vi "AutonomousMain.vi"() -> (0 "Terminate":bool)   [LabVIEW 2015]
uses:
  <vilib>/Rock Robotics/WPI/DriverStation/WPI_DriverStationRobotMode2.ctl
  <vilib>/Rock Robotics/WPI/CAN/TalonSRX/WPI_CANTalonSRX_APIControlMode.ctl
  <vilib>/Rock Robotics/WPI/Solenoid/WPI_SolenoidValue.ctl
  Utilities/AutoVars.vi
  Utilities/MotorPositionGlobals.vi
  Utilities/GlobalVisionVars.vi
  Utilities/VisionGlobals.vi
  <vilib>/Rock Robotics/WPI/Solenoid/WPI_SolenoidSetEnum.vi
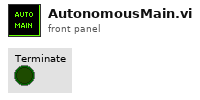
[diagram p1: front panel]
types:
  T1 = enum16{"WaitingForInput", "Driving", "TurnToTarget", "DriveMore", "Shoot", "End"}
  T2 = typedef "WPI_DriverStationRobotMode2.ctl" = enum16{"Autonomous Disabled", "Autonomous Enabled", "Teleop Disabled", "Teleop Enabled", "Disconnected", "Finish", "Test Disabled", "Test Enabled", "Emergency Stopped"}
  T3 = enum16{"Far Left", "Pos 2", "Pos 3", "Pos 4", "Far Right"}
  T4 = typedef "WPI_SolenoidValue.ctl" = enum16{"Off", "On", "Forward", "Reverse"}
  T5 = typedef "WPI_MotorControlDeviceRef.ctl" = cluster{"DeviceStatus":errorcluster, "Type":T6, "PWM":cluster{"PWM Channel":T7, "DeadBand":T8}, "CAN":cluster{"Device Number":u8, "Control Mode":T9, "Semaphore":T10, "Max Vout":dbl, "TalonSRX Control Mode":T11}, "Invert":bool}
  T6 = typedef "WPI_MotorControlType.ctl" = enum16{"PWM", "CAN", "CANTalonSRX"}
  T7 = typedef "FPGA_DIOPWMChannel.ctl" = enum8{"PWM 0", "PWM 1", "PWM 2", "PWM 3", "PWM 4", "PWM 5", "PWM 6", "PWM 7", "PWM 8", "PWM 9", "PWM MXP 0", "PWM MXP 1", "PWM MXP 2", "PWM MXP 3", "PWM MXP 4", "PWM MXP 5", "PWM MXP 6", "PWM MXP 7", "PWM MXP 8", "PWM MXP 9", "Invalid"}
  T8 = typedef "WPI_PWMDeadband.ctl" = cluster{"Name":string, "maxPositivePwm":i32, "minPositivePwm":i32, "centerPwm":i32, "maxNegativePwm":i32, "minNegativePwm":i32, "angularRange":u16}
  T9 = typedef "WPI_CANJaguar_ControlMode.ctl" = enum8{"Percent VBus", "Current", "Speed", "Position", "Voltage"}
  T10 = typedef "Semaphore RefNum" = refnum<k1>
  T11 = typedef "WPI_CANTalonSRX_APIControlMode.ctl" = enum8{"Percent VBus", "Speed", "Position", "Slave", "Unchanged / Invalid", "Voltage Compensation", "Current", "Motion Profile"}
  T12 = typedef "WPI_DigitalOutputDevRef.ctl" = cluster{"DIO Channel":T13, "DevStatus":errorcluster}
  T13 = typedef "FPGA_DIOChannel.ctl" = enum8{"DIO 0", "DIO 1", "DIO 2", "DIO 3", "DIO 4", "DIO 5", "DIO 6", "DIO 7", "DIO 8", "DIO 9", "DIO MXP 0", "DIO MXP 1", "DIO MXP 2", "DIO MXP 3", "DIO MXP 4", "DIO MXP 5", "DIO MXP 6", "DIO MXP 7", "DIO MXP 8", "DIO MXP 9", "DIO MXP 10", "DIO MXP 11", "DIO MXP 12", "DIO MXP 13", "DIO MXP 14", "DIO MXP 15", "Invalid"}
  T14 = typedef "WPI_GyroDevRef.ctl" = cluster{"DevStatus":errorcluster, "Analog Channel":T15, "Offset":dbl, "Gain (VoltsPerDegree/Second)":dbl, "Gyro Type":enum16{"Analog", "XRS450"}, "Handle":i32, "SPI Bus":T16, "Device Found":bool, "Sample Rate":dbl, "Calibrate On Open":bool}
  T15 = typedef "FPGA_AIChannel.ctl" = enum8{"AI 0", "AI 1", "AI 2", "AI 3", "AI MXP 0", "AI MXP 1", "AI MXP 2", "AI MXP 3", "Invalid"}
  T16 = typedef "spi_bus.ctl" = enum16{"SPI On-Board, CS0", "SPI On-Board, CS1", "SPI On-Board, CS2", "SPI On-Board, CS3", "SPI MXP", "Invalid"}
  T17 = typedef "WPI_SolenoidDevRef.ctl" = cluster{"DevStatus":errorcluster, "Pneumatics Control Module":u8, "Forward Solenoid Channel":T18, "Reverse Solenoid Channel":T18}
  T18 = typedef "WPI_SolenoidChannel.ctl" = enum8{"Solenoid 0", "Solenoid 1", "Solenoid 2", "Solenoid 3", "Solenoid 4", "Solenoid 5", "Solenoid 6", "Solenoid 7", "Invalid"}
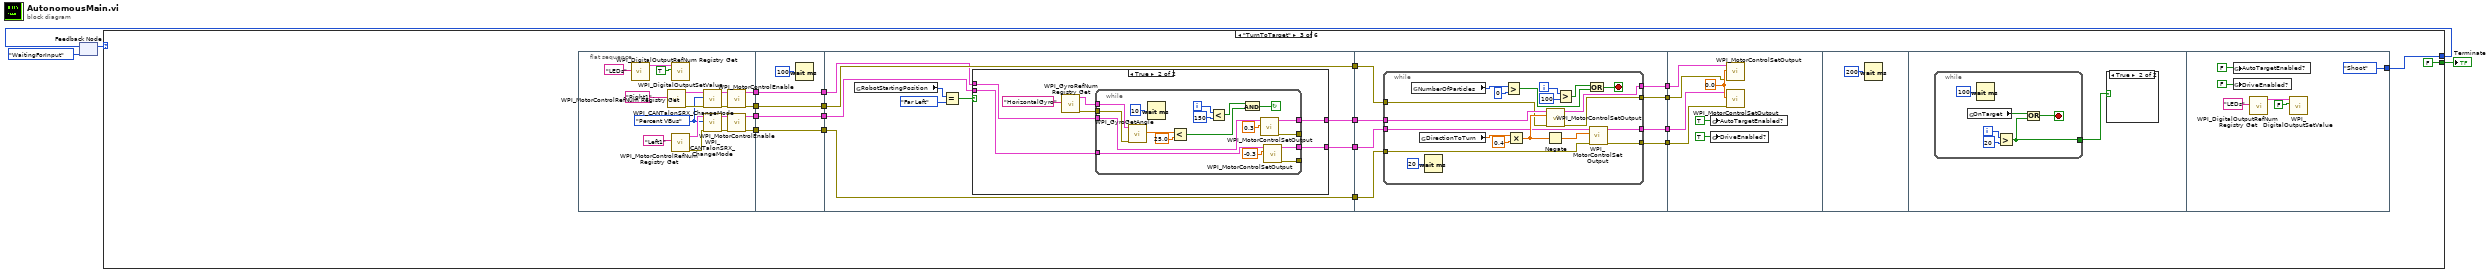
[diagram p0: block diagram]
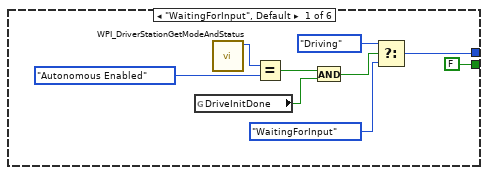
[diagram p2: hidden frame]
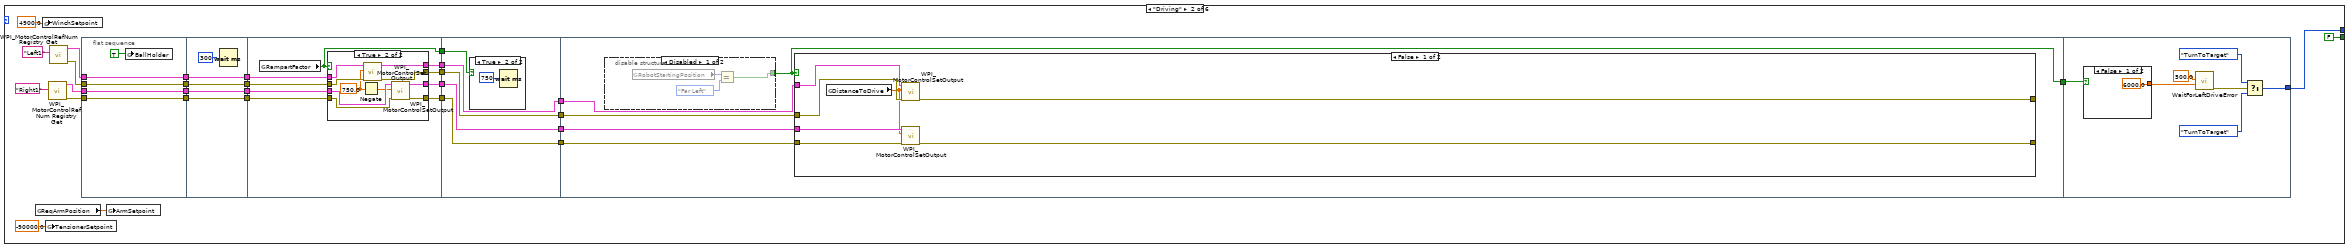
[diagram p3: hidden frame]
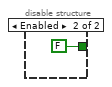
[diagram p6: hidden frame]
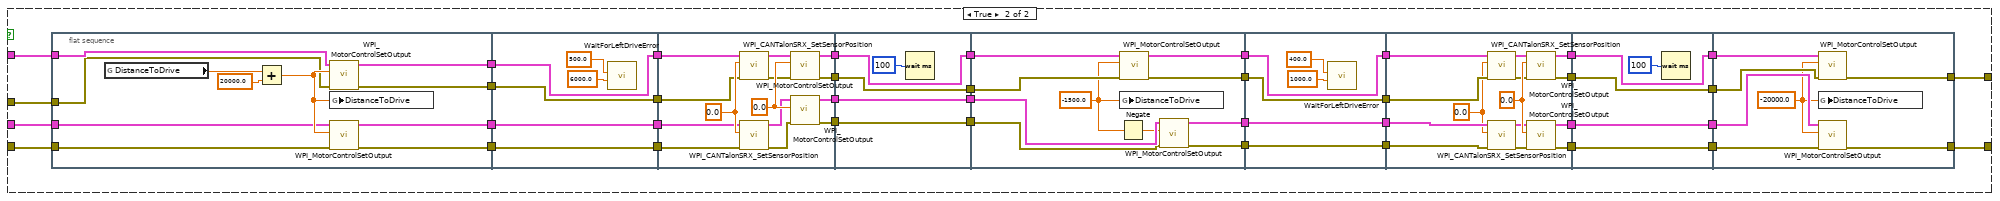
[diagram p7: hidden frame]
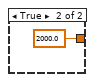
[diagram p8: hidden frame]
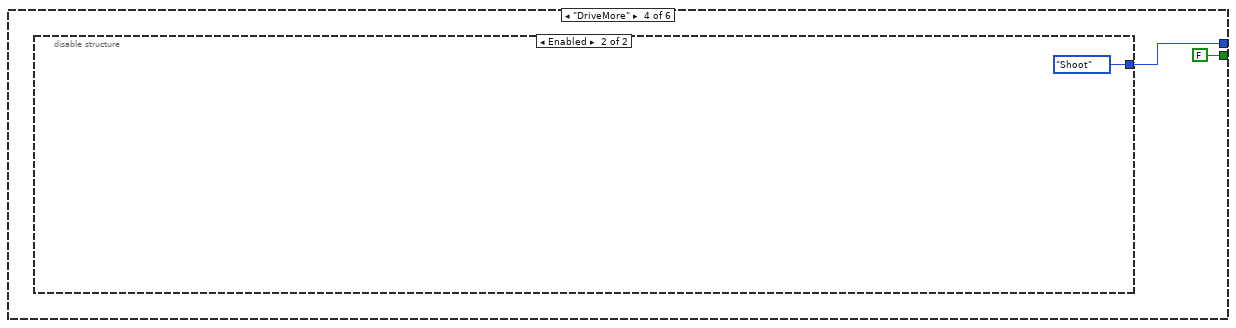
[diagram p11: hidden frame]
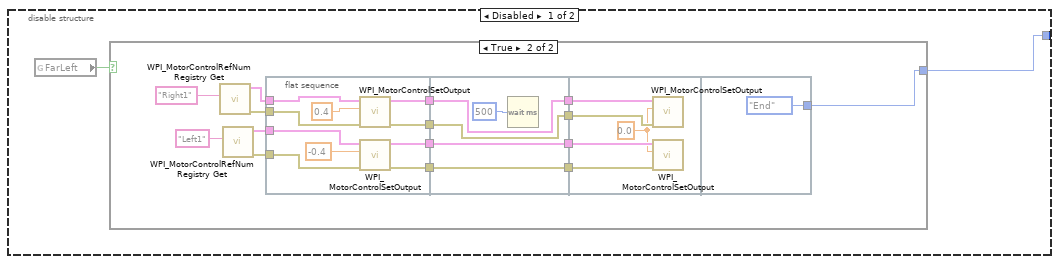
[diagram p12: hidden frame]
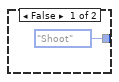
[diagram p13: hidden frame]
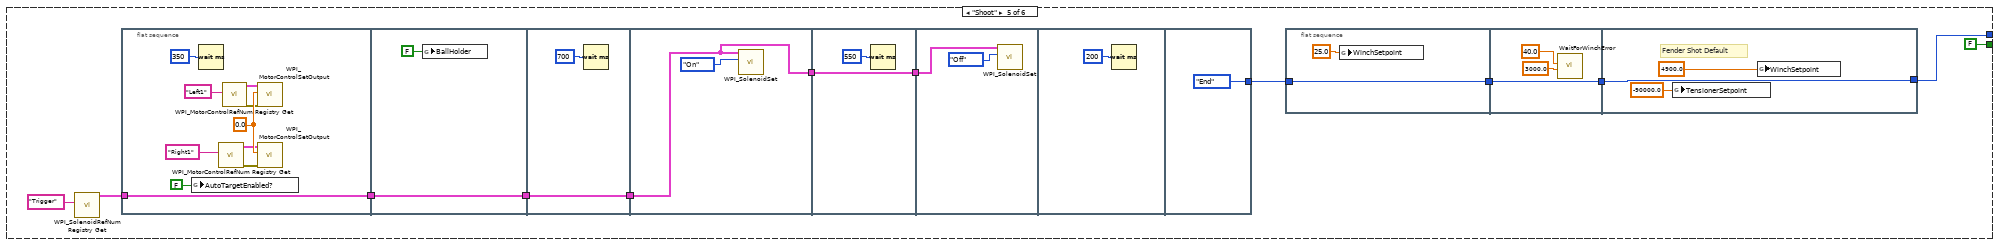
[diagram p14: hidden frame]
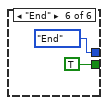
[diagram p15: hidden frame]
diagram:
  n1 = feedback #1(T1."WaitingForInput" ("AutoStateMachine")) -> (w1:T1)
  n2 = case shown="\"TurnToTarget\"" w1 {
    tunnel: [w13 w25 w240 w350 w393 T1."End" ("AutoStateMachine")] -> w4
    tunnel: [FALSE FALSE FALSE FALSE FALSE TRUE] -> w3
    frame "WaitingForInput", Default {
      n3 = global read "AutoVars.vi" "DriveInitDone"() -> (w8:bool)
      n4 = call <vilib>:"WPI_DriverStationGetModeAndStatus.vi"() -> ("Robot Mode"=w11:T2)  [unwired: 10 in, 1 out]
      n5 = Equal?(x=w11, y=WPI_DriverStationRobotMode2."Autonomous Enabled" ("Robot Mode")) -> (x = y?=w9:bool)
      n6 = And(x=w9, y=w8) -> (x .and. y?=w7:bool)
      n7 = Select(t=T1."Driving" ("AutoStateMachine"), s=w7, f=T1."WaitingForInput" ("AutoStateMachine")) -> (s? t:f=w13:T1)
    }
    frame "Driving" {
      n8 = global read "AutoVars.vi" "ReqArmPosition"() -> (w24:dbl)
      n9 = global write "MotorPositionGlobals.vi" "WinchSetpoint"(4900.0 ("WinchSetpoint")) -> ()
      n10 = global write "MotorPositionGlobals.vi" "TensionerSetpoint"(-90000.0 ("TensionerSetpoint")) -> ()
      n11 = call <vilib>:"WPI_MotorControlRefNum Registry Get.vi"("refnum name"="Right1") -> ("error out"=w36:errorcluster, "MotorControlDevRef"=w37:T5)  [unwired: 9 in]
      n12 = call <vilib>:"WPI_MotorControlRefNum Registry Get.vi"("refnum name"="Left1") -> ("error out"=w34:errorcluster, "MotorControlDevRef"=w35:T5)  [unwired: 9 in]
      n13 = flat-sequence {
        tunnel: w34 -> [w44]
        tunnel: w35 -> [w45]
        tunnel: w36 -> [w46]
        tunnel: w37 -> [w47]
        tunnel: [w47] -> w23
        tunnel: [w46] -> w21
        tunnel: [w45] -> w19
        tunnel: [w44] -> w17
        tunnel: w23 -> [w52]
        tunnel: [w52] -> w22
        tunnel: w21 -> [w51]
        tunnel: [w51] -> w20
        tunnel: w19 -> [w50]
        tunnel: [w50] -> w18
        tunnel: w17 -> [w49]
        tunnel: [w49] -> w16
        tunnel: [w57] -> w33
        tunnel: [w56] -> w31
        tunnel: [w55] -> w29
        tunnel: [w54] -> w27
        tunnel: w22 -> [w61]
        tunnel: w20 -> [w60]
        tunnel: w18 -> [w59]
        tunnel: w16 -> [w58]
        tunnel: [w53] -> w15
        tunnel: w33 -> [w80]
        tunnel: [w80] -> w32
        tunnel: w31 -> [w79]
        tunnel: [w79] -> w30
        tunnel: w29 -> [w78]
        tunnel: [w78] -> w28
        tunnel: w27 -> [w77]
        tunnel: [w77] -> w26
        tunnel: w15 -> [w76]
        tunnel: w32 -> [w86]
        tunnel: w30 -> [w85]
        tunnel: w28 -> [w83]
        tunnel: w26 -> [w84]
        tunnel: [w82] -> w14
        tunnel: [w215] -> w25
        tunnel: w14 -> [w214]
        frame #0 {
          n14 = global write "MotorPositionGlobals.vi" "BallHolder"(TRUE ("BallHolder")) -> ()
        }
        frame #1 {
          n15 = Wait (ms)(milliseconds to wait=u32 300) -> ()  [unwired: 1 out]
        }
        frame #2 {
          n16 = global read "AutoVars.vi" "RampartFactor"() -> (w53:bool)
          n17 = case shown="True" w53 {
            tunnel: w61 -> [w63 w75]
            tunnel: w60 -> [w62 w74]
            tunnel: w59 -> [w65 w73]
            tunnel: w58 -> [w64 w72]
            tunnel: [w63 w71] -> w57
            tunnel: [w62 w70] -> w56
            tunnel: [w65 w69] -> w55
            tunnel: [w64 w68] -> w54
            frame False {
            }
            frame True {
              w67 = 750.0
              n18 = Negate(x=w67) -> (-x=w66:dbl)
              n19 = call <vilib>:"WPI_MotorControlSetOutput.vi"("error in (no error)"=w72, "Output"=w67, "MotorControlDevRef"=w73) -> ("error out"=w68:errorcluster, "MotorControlDevRef"=w69:T5)  [unwired: 6 in, 1 out]
              n20 = call <vilib>:"WPI_MotorControlSetOutput.vi"("error in (no error)"=w74, "Output"=w66, "MotorControlDevRef"=w75) -> ("error out"=w70:errorcluster, "MotorControlDevRef"=w71:T5)  [unwired: 6 in, 1 out]
            }
          }
        }
        frame #3 {
          n21 = case shown="True" w76 {
            frame False {
            }
            frame True {
              n22 = Wait (ms)(milliseconds to wait=u32 750) -> ()  [unwired: 1 out]
            }
          }
        }
        frame #4 {
          n23 = disable-structure shown="Disabled" {
            disable-tunnel: [w87 FALSE] -> w82
            frame Disabled {
              n24 = global read "AutoVars.vi" "RobotStartingPosition"() -> (w89:T3)
              n25 = Equal?(x=w89, y=T3."Far Left") -> (x = y?=w87:bool)
            }
            frame Enabled {
            }
          }
          n26 = case shown="False" w82 {
            tunnel: w86 -> [w97 w134]
            tunnel: w85 -> [w96 w132]
            tunnel: w84 -> [w95 w133]
            tunnel: w83 -> [w93 w135]
            tunnel: [w92 w115] -> _
            tunnel: [w91 w114] -> _
            frame False {
              n27 = global read "AutoVars.vi" "DistanceToDrive"() -> (w94:dbl)
              n28 = call <vilib>:"WPI_MotorControlSetOutput.vi"("error in (no error)"=w95, "Output"=w94, "MotorControlDevRef"=w93) -> ("error out"=w92:errorcluster)  [unwired: 6 in, 2 out]
              n29 = call <vilib>:"WPI_MotorControlSetOutput.vi"("error in (no error)"=w96, "Output"=w94, "MotorControlDevRef"=w97) -> ("error out"=w91:errorcluster)  [unwired: 6 in, 2 out]
            }
            frame True {
              n30 = flat-sequence {
                tunnel: w135 -> [w143]
                tunnel: w134 -> [w142]
                tunnel: w133 -> [w141]
                tunnel: w132 -> [w140]
                tunnel: [w139] -> w130
                tunnel: [w138] -> w128
                tunnel: [w137] -> w126
                tunnel: [w136] -> w125
                tunnel: [w150] -> w131
                tunnel: w130 -> [w150]
                tunnel: [w149] -> w129
                tunnel: w128 -> [w149]
                tunnel: [w148] -> w127
                tunnel: w126 -> [w148]
                tunnel: w125 -> [w147]
                tunnel: [w147] -> w124
                tunnel: w131 -> [w160]
                tunnel: w129 -> [w159]
                tunnel: w127 -> [w158]
                tunnel: w124 -> [w157]
                tunnel: [w156] -> w113
                tunnel: [w155] -> w111
                tunnel: [w154] -> w109
                tunnel: [w153] -> w107
                tunnel: w113 -> [w171]
                tunnel: [w171] -> w112
                tunnel: w111 -> [w170]
                tunnel: [w170] -> w110
                tunnel: w109 -> [w169]
                tunnel: [w169] -> w108
                tunnel: w107 -> [w168]
                tunnel: [w168] -> w106
                tunnel: w112 -> [w181]
                tunnel: w110 -> [w180]
                tunnel: w108 -> [w179]
                tunnel: w106 -> [w178]
                tunnel: [w177] -> w123
                tunnel: [w176] -> w121
                tunnel: [w175] -> w119
                tunnel: [w174] -> w117
                tunnel: w123 -> [w187]
                tunnel: [w187] -> w122
                tunnel: w121 -> [w186]
                tunnel: [w186] -> w120
                tunnel: w119 -> [w185]
                tunnel: [w185] -> w118
                tunnel: w117 -> [w184]
                tunnel: [w184] -> w116
                tunnel: w122 -> [w200]
                tunnel: w120 -> [w199]
                tunnel: w118 -> [w198]
                tunnel: w116 -> [w197]
                tunnel: [w195] -> w99
                tunnel: [w194] -> w101
                tunnel: [w193] -> w103
                tunnel: [w192] -> w105
                tunnel: w105 -> [w206]
                tunnel: [w206] -> w104
                tunnel: w103 -> [w205]
                tunnel: [w205] -> w102
                tunnel: w101 -> [w204]
                tunnel: [w204] -> w100
                tunnel: w99 -> [w203]
                tunnel: [w203] -> w98
                tunnel: w104 -> [w210]
                tunnel: w102 -> [w211]
                tunnel: w100 -> [w212]
                tunnel: w98 -> [w213]
                tunnel: [w209] -> w115
                tunnel: [w208] -> w114
                frame #0 {
                  n31 = global read "AutoVars.vi" "DistanceToDrive"() -> (w145:dbl)
                  n32 = Add(x=w145, y=20000.0) -> (x+y=w144:dbl)
                  n33 = call <vilib>:"WPI_MotorControlSetOutput.vi"("error in (no error)"=w141, "Output"=w144, "MotorControlDevRef"=w143) -> ("error out"=w138:errorcluster, "MotorControlDevRef"=w139:T5)  [unwired: 6 in, 1 out]
                  n34 = global write "AutoVars.vi" "DistanceToDrive"(w144) -> ()
                  n35 = call <vilib>:"WPI_MotorControlSetOutput.vi"("error in (no error)"=w140, "Output"=w144, "MotorControlDevRef"=w142) -> ("error out"=w136:errorcluster, "MotorControlDevRef"=w137:T5)  [unwired: 6 in, 1 out]
                }
                frame #1 {
                  n36 = call "WaitForLeftDriveError.vi"("Timeout (ms)"=6000.0, "AllowedError"=500.0) -> ()  [unwired: 9 in, 1 out]
                }
                frame #2 {
                  w165 = 0.0 ("New Sensor Position")
                  w166 = 0.0 ("Output")
                  n37 = call <vilib>:"WPI_CANTalonSRX_SetSensorPosition.vi"("error in (no error)"=w159, "New Sensor Position"=w165, "CAN Talon SRX Ref"=w160) -> ("error out"=w163:errorcluster, "CAN Talon SRX Ref"=w164:T5)  [unwired: 7 in]
                  n38 = call <vilib>:"WPI_CANTalonSRX_SetSensorPosition.vi"("error in (no error)"=w157, "New Sensor Position"=w165, "CAN Talon SRX Ref"=w158) -> ("error out"=w161:errorcluster, "CAN Talon SRX Ref"=w162:T5)  [unwired: 7 in]
                  n39 = call <vilib>:"WPI_MotorControlSetOutput.vi"("error in (no error)"=w163, "Output"=w166, "MotorControlDevRef"=w164) -> ("error out"=w155:errorcluster, "MotorControlDevRef"=w156:T5)  [unwired: 6 in, 1 out]
                  n40 = call <vilib>:"WPI_MotorControlSetOutput.vi"("error in (no error)"=w161, "Output"=w166, "MotorControlDevRef"=w162) -> ("error out"=w153:errorcluster, "MotorControlDevRef"=w154:T5)  [unwired: 6 in, 1 out]
                }
                frame #3 {
                  n41 = Wait (ms)(milliseconds to wait=u32 100) -> ()  [unwired: 1 out]
                }
                frame #4 {
                  w172 = -1500.0
                  n42 = Negate(x=w172) -> (-x=w173:dbl)
                  n43 = call <vilib>:"WPI_MotorControlSetOutput.vi"("error in (no error)"=w180, "Output"=w172, "MotorControlDevRef"=w181) -> ("error out"=w176:errorcluster, "MotorControlDevRef"=w177:T5)  [unwired: 6 in, 1 out]
                  n44 = global write "AutoVars.vi" "DistanceToDrive"(w172) -> ()
                  n45 = call <vilib>:"WPI_MotorControlSetOutput.vi"("error in (no error)"=w178, "Output"=w173, "MotorControlDevRef"=w179) -> ("error out"=w174:errorcluster, "MotorControlDevRef"=w175:T5)  [unwired: 6 in, 1 out]
                }
                frame #5 {
                  n46 = call "WaitForLeftDriveError.vi"("Timeout (ms)"=1000.0, "AllowedError"=400.0) -> ()  [unwired: 9 in, 1 out]
                }
                frame #6 {
                  w196 = 0.0 ("New Sensor Position")
                  w201 = 0.0 ("Output")
                  n47 = call <vilib>:"WPI_CANTalonSRX_SetSensorPosition.vi"("error in (no error)"=w199, "New Sensor Position"=w196, "CAN Talon SRX Ref"=w200) -> ("error out"=w190:errorcluster, "CAN Talon SRX Ref"=w191:T5)  [unwired: 7 in]
                  n48 = call <vilib>:"WPI_CANTalonSRX_SetSensorPosition.vi"("error in (no error)"=w197, "New Sensor Position"=w196, "CAN Talon SRX Ref"=w198) -> ("error out"=w188:errorcluster, "CAN Talon SRX Ref"=w189:T5)  [unwired: 7 in]
                  n49 = call <vilib>:"WPI_MotorControlSetOutput.vi"("error in (no error)"=w190, "Output"=w201, "MotorControlDevRef"=w191) -> ("error out"=w194:errorcluster, "MotorControlDevRef"=w195:T5)  [unwired: 6 in, 1 out]
                  n50 = call <vilib>:"WPI_MotorControlSetOutput.vi"("error in (no error)"=w188, "Output"=w201, "MotorControlDevRef"=w189) -> ("error out"=w192:errorcluster, "MotorControlDevRef"=w193:T5)  [unwired: 6 in, 1 out]
                }
                frame #7 {
                  n51 = Wait (ms)(milliseconds to wait=u32 100) -> ()  [unwired: 1 out]
                }
                frame #8 {
                  w207 = -20000.0 ("Output")
                  n52 = call <vilib>:"WPI_MotorControlSetOutput.vi"("error in (no error)"=w212, "Output"=w207, "MotorControlDevRef"=w213) -> ("error out"=w209:errorcluster)  [unwired: 6 in, 2 out]
                  n53 = global write "AutoVars.vi" "DistanceToDrive"(w207) -> ()
                  n54 = call <vilib>:"WPI_MotorControlSetOutput.vi"("error in (no error)"=w210, "Output"=w207, "MotorControlDevRef"=w211) -> ("error out"=w208:errorcluster)  [unwired: 6 in, 2 out]
                }
              }
            }
          }
        }
        frame #5 {
          n55 = case shown="False" w214 {
            tunnel: [6000.0 ("Timeout (ms)") 2000.0 ("Timeout (ms)")] -> w220
            frame False {
            }
            frame True {
            }
          }
          n56 = call "WaitForLeftDriveError.vi"("Timeout (ms)"=w220, "AllowedError"=500.0) -> ("error out"=w218:errorcluster)  [unwired: 9 in]
          n57 = Select(t=T1."TurnToTarget", s=w218, f=T1."TurnToTarget" ("AutoStateMachine")) -> (s? t:f=w215:T1)
        }
      }
      n58 = global write "MotorPositionGlobals.vi" "ArmSetpoint"(w24) -> ()
    }
    frame "TurnToTarget" {
      n59 = flat-sequence {
        tunnel: [w247] -> w238
        tunnel: [w246] -> w237
        tunnel: [w245] -> w236
        tunnel: [w244] -> w235
        tunnel: w238 -> [w260]
        tunnel: w237 -> [w259]
        tunnel: w236 -> [w262]
        tunnel: w235 -> [w261]
        tunnel: [w262] -> w230
        tunnel: [w261] -> w228
        tunnel: [w260] -> w226
        tunnel: [w259] -> w224
        tunnel: w230 -> [w267]
        tunnel: [w266] -> w229
        tunnel: w228 -> [w272]
        tunnel: [w272] -> w227
        tunnel: w226 -> [w265]
        tunnel: [w264] -> w225
        tunnel: w224 -> [w271]
        tunnel: [w271] -> w223
        tunnel: [w307] -> w234
        tunnel: [w306] -> w233
        tunnel: [w305] -> w232
        tunnel: [w304] -> w231
        tunnel: w229 -> [w303]
        tunnel: w227 -> [w302]
        tunnel: w225 -> [w301]
        tunnel: w223 -> [w300]
        tunnel: w234 -> [w331]
        tunnel: w233 -> [w330]
        tunnel: w232 -> [w329]
        tunnel: w231 -> [w328]
        tunnel: [T1."Shoot" ("AutoStateMachine")] -> w240
        frame #0 {
          w252 = WPI_CANTalonSRX_APIControlMode."Percent VBus" ("Control Mode")
          n60 = call <vilib>:"WPI_DigitalOutputRefNum Registry Get.vi"("refnum name"="LEDs") -> ("DigitalOutputDevRef"=w242:T12)  [unwired: 9 in, 1 out]
          n61 = call <vilib>:"WPI_MotorControlRefNum Registry Get.vi"("refnum name"="Right1") -> ("error out"=w256:errorcluster, "MotorControlDevRef"=w255:T5)  [unwired: 9 in]
          n62 = call <vilib>:"WPI_MotorControlRefNum Registry Get.vi"("refnum name"="Left1") -> ("error out"=w254:errorcluster, "MotorControlDevRef"=w253:T5)  [unwired: 9 in]
          n63 = call <vilib>:"WPI_DigitalOutputSetValue.vi"("Value"=TRUE, "DigitalOutputDevRef"=w242) -> ()  [unwired: 8 in, 2 out]
          n64 = call <vilib>:"WPI_CANTalonSRX_ChangeMode.vi"("error in (no error)"=w256, "Control Mode"=w252, "CAN Talon SRX Ref"=w255) -> ("error out"=w250:errorcluster, "CAN Talon SRX Ref"=w251:T5)  [unwired: 7 in]
          n65 = call <vilib>:"WPI_CANTalonSRX_ChangeMode.vi"("error in (no error)"=w254, "Control Mode"=w252, "CAN Talon SRX Ref"=w253) -> ("error out"=w248:errorcluster, "CAN Talon SRX Ref"=w249:T5)  [unwired: 7 in]
          n66 = call <vilib>:"WPI_MotorControlEnable.vi"("error in (no error)"=w250, "CAN MotorDevRef"=w251) -> ("error out"=w244:errorcluster, "CAN MotorDevRef"=w245:T5)  [unwired: 8 in]
          n67 = call <vilib>:"WPI_MotorControlEnable.vi"("error in (no error)"=w248, "CAN MotorDevRef"=w249) -> ("error out"=w246:errorcluster, "CAN MotorDevRef"=w247:T5)  [unwired: 8 in]
        }
        frame #1 {
          n68 = Wait (ms)(milliseconds to wait=u32 100) -> ()  [unwired: 1 out]
        }
        frame #2 {
          n69 = global read "AutoVars.vi" "RobotStartingPosition"() -> (w270:T3)
          n70 = Equal?(x=w270, y=T3."Far Left") -> (x = y?=w268:bool)
          n71 = case shown="True" w268 {
            tunnel: w267 -> [w274 w281]
            tunnel: [w274 w280] -> w266
            tunnel: w265 -> [w273 w279]
            tunnel: [w273 w278] -> w264
            frame False {
            }
            frame True {
              n72 = call <vilib>:"WPI_GyroRefNum Registry Get.vi"("refnum name"="HorizontalGyro") -> ("error out"=w275:errorcluster, "GyroDevRef"=w276:T14)  [unwired: 9 in]
              n73 = while {
                tunnel: w279 -> [w297]
                tunnel: w281 -> [w296]
                tunnel: [w295] -> w278
                tunnel: [w294] -> _
                tunnel: [w293] -> w280
                tunnel: [w292] -> _
                tunnel: w276 -> [w291]
                tunnel: w275 -> [w290]
                i -> [w283]
                stop <- w286 continue-if-true
                n74 = call <vilib>:"WPI_GyroGetAngle.vi"("error in"=w290, "GyroDevRef"=w291) -> ("Angle"=w289:dbl)  [unwired: 5 in, 4 out]
                n75 = Wait (ms)(milliseconds to wait=u32 10) -> ()  [unwired: 1 out]
                n76 = Less?(x=w289, y=25.0) -> (x < y?=w285:bool)
                n77 = Less?(x=w283, y=150) -> (x < y?=w284:bool)
                n78 = And(x=w284, y=w285) -> (x .and. y?=w286:bool)
                n79 = call <vilib>:"WPI_MotorControlSetOutput.vi"("Output"=0.3, "MotorControlDevRef"=w296) -> ("error out"=w292:errorcluster, "MotorControlDevRef"=w293:T5)  [unwired: 7 in, 1 out]
                n80 = call <vilib>:"WPI_MotorControlSetOutput.vi"("Output"=-0.3, "MotorControlDevRef"=w297) -> ("error out"=w294:errorcluster, "MotorControlDevRef"=w295:T5)  [unwired: 7 in, 1 out]
              }
            }
          }
        }
        frame #3 {
          n81 = while {
            tunnel: [w320] -> w307
            tunnel: [w319] -> w306
            tunnel: [w318] -> w305
            tunnel: [w317] -> w304
            tunnel: w303 -> [w316]
            tunnel: w302 -> [w315]
            tunnel: w301 -> [w314]
            tunnel: w300 -> [w313]
            i -> [w309]
            stop <- w312 stop-if-true
            n82 = global read "GlobalVisionVars.vi" "NumberOfParticles"() -> (w327:i32)
            n83 = global read "AutoVars.vi" "DirectionToTurn"() -> (w324:dbl)
            n84 = Wait (ms)(milliseconds to wait=u32 20) -> ()  [unwired: 1 out]
            n85 = Greater?(x=w327, y=0) -> (0:w311:bool)
            n86 = Multiply(x=w324, y=0.4) -> (x*y=w321:dbl)
            n87 = Negate(x=w321) -> (-x=w322:dbl)
            n88 = call <vilib>:"WPI_MotorControlSetOutput.vi"("error in (no error)"=w315, "Output"=w321, "MotorControlDevRef"=w316) -> ("error out"=w319:errorcluster, "MotorControlDevRef"=w320:T5)  [unwired: 6 in, 1 out]
            n89 = Greater?(x=w309, y=100) -> (0:w310:bool)
            n90 = Or(x=w310, y=w311) -> (x .or. y?=w312:bool)
            n91 = call <vilib>:"WPI_MotorControlSetOutput.vi"("error in (no error)"=w313, "Output"=w322, "MotorControlDevRef"=w314) -> ("error out"=w317:errorcluster, "MotorControlDevRef"=w318:T5)  [unwired: 6 in, 1 out]
          }
        }
        frame #4 {
          w333 = 0.0
          n92 = global write "VisionGlobals.vi" "AutoTargetEnabled?"(TRUE ("AutoTargetEnabled?")) -> ()
          n93 = global write "VisionGlobals.vi" "DriveEnabled?"(TRUE ("DriveEnabled?")) -> ()
          n94 = call <vilib>:"WPI_MotorControlSetOutput.vi"("error in (no error)"=w330, "Output"=w333, "MotorControlDevRef"=w331) -> ()  [unwired: 6 in, 3 out]
          n95 = call <vilib>:"WPI_MotorControlSetOutput.vi"("error in (no error)"=w328, "Output"=w333, "MotorControlDevRef"=w329) -> ()  [unwired: 6 in, 3 out]
        }
        frame #5 {
          n96 = Wait (ms)(milliseconds to wait=u32 200) -> ()  [unwired: 1 out]
        }
        frame #6 {
          n97 = while {
            tunnel: [w337] -> w336
            i -> [w339]
            stop <- w340 stop-if-true
            n98 = global read "GlobalVisionVars.vi" "OnTarget"() -> (w341:bool)
            n99 = Wait (ms)(milliseconds to wait=u32 100) -> ()  [unwired: 1 out]
            n100 = Greater?(x=w339, y=20) -> (0:w337:bool)
            n101 = Or(x=w341, y=w337) -> (x .or. y?=w340:bool)
          }
          n102 = case shown="True" w336 {
            frame False {
            }
            frame True {
            }
          }
        }
        frame #7 {
          n103 = global write "VisionGlobals.vi" "AutoTargetEnabled?"(FALSE ("AutoTargetEnabled?")) -> ()
          n104 = global write "VisionGlobals.vi" "DriveEnabled?"(FALSE ("DriveEnabled?")) -> ()
          n105 = call <vilib>:"WPI_DigitalOutputRefNum Registry Get.vi"("refnum name"="LEDs") -> ("DigitalOutputDevRef"=w346:T12)  [unwired: 9 in, 1 out]
          n106 = call <vilib>:"WPI_DigitalOutputSetValue.vi"("Value"=FALSE, "DigitalOutputDevRef"=w346) -> ()  [unwired: 8 in, 2 out]
        }
      }
    }
    frame "DriveMore" {
      n107 = disable-structure shown="Enabled" {
        disable-tunnel: [w352 T1."Shoot" ("AutoStateMachine")] -> w350
        frame Disabled {
          n108 = global read "AutoVars.vi" "FarLeft"() -> (w351:bool)
          n109 = case shown="True" w351 {
            tunnel: [T1."Shoot" ("AutoStateMachine") w366] -> w352
            frame False {
            }
            frame True {
              n110 = call <vilib>:"WPI_MotorControlRefNum Registry Get.vi"("refnum name"="Right1") -> ("error out"=w362:errorcluster, "MotorControlDevRef"=w363:T5)  [unwired: 9 in]
              n111 = call <vilib>:"WPI_MotorControlRefNum Registry Get.vi"("refnum name"="Left1") -> ("error out"=w364:errorcluster, "MotorControlDevRef"=w365:T5)  [unwired: 9 in]
              n112 = flat-sequence {
                tunnel: w365 -> [w378]
                tunnel: w364 -> [w377]
                tunnel: w363 -> [w376]
                tunnel: w362 -> [w375]
                tunnel: [w374] -> w361
                tunnel: [w373] -> w360
                tunnel: [w372] -> w359
                tunnel: [w371] -> w355
                tunnel: w361 -> [w381]
                tunnel: w360 -> [w379]
                tunnel: w359 -> [w382]
                tunnel: [w382] -> w358
                tunnel: [w381] -> w357
                tunnel: [w380] -> w356
                tunnel: w355 -> [w380]
                tunnel: [w379] -> w354
                tunnel: w358 -> [w388]
                tunnel: w357 -> [w387]
                tunnel: w356 -> [w386]
                tunnel: w354 -> [w385]
                tunnel: [T1."End" ("AutoStateMachine")] -> w366
                frame #0 {
                  n113 = call <vilib>:"WPI_MotorControlSetOutput.vi"("error in (no error)"=w375, "Output"=0.4, "MotorControlDevRef"=w376) -> ("error out"=w374:errorcluster, "MotorControlDevRef"=w372:T5)  [unwired: 6 in, 1 out]
                  n114 = call <vilib>:"WPI_MotorControlSetOutput.vi"("error in (no error)"=w377, "Output"=-0.4, "MotorControlDevRef"=w378) -> ("error out"=w373:errorcluster, "MotorControlDevRef"=w371:T5)  [unwired: 6 in, 1 out]
                }
                frame #1 {
                  n115 = Wait (ms)(milliseconds to wait=u32 500) -> ()  [unwired: 1 out]
                }
                frame #2 {
                  w384 = 0.0 ("Output")
                  n116 = call <vilib>:"WPI_MotorControlSetOutput.vi"("error in (no error)"=w387, "Output"=w384, "MotorControlDevRef"=w388) -> ()  [unwired: 6 in, 3 out]
                  n117 = call <vilib>:"WPI_MotorControlSetOutput.vi"("error in (no error)"=w385, "Output"=w384, "MotorControlDevRef"=w386) -> ()  [unwired: 6 in, 3 out]
                }
                frame #3 {
                }
              }
            }
          }
        }
        frame Enabled {
        }
      }
    }
    frame "Shoot" {
      n118 = call <vilib>:"WPI_SolenoidRefNum Registry Get.vi"("refnum name"="Trigger") -> ("SolenoidDevRef"=w398:T17)  [unwired: 9 in, 1 out]
      n119 = flat-sequence {
        tunnel: [w420] -> w392
        tunnel: w398 -> [w420]
        tunnel: w392 -> [w422]
        tunnel: [w422] -> w391
        tunnel: w391 -> [w424]
        tunnel: [w424] -> w402
        tunnel: [w425] -> w401
        tunnel: w402 -> [w425]
        tunnel: w401 -> [w427]
        tunnel: [w427] -> w400
        tunnel: w400 -> [w429]
        tunnel: [T1."End" ("AutoStateMachine")] -> w396
        frame #0 {
          w415 = 0.0
          n120 = global write "VisionGlobals.vi" "AutoTargetEnabled?"(FALSE ("AutoTargetEnabled?")) -> ()
          n121 = Wait (ms)(milliseconds to wait=u32 350) -> ()  [unwired: 1 out]
          n122 = call <vilib>:"WPI_MotorControlRefNum Registry Get.vi"("refnum name"="Right1") -> ("error out"=w413:errorcluster, "MotorControlDevRef"=w414:T5)  [unwired: 9 in]
          n123 = call <vilib>:"WPI_MotorControlRefNum Registry Get.vi"("refnum name"="Left1") -> ("error out"=w411:errorcluster, "MotorControlDevRef"=w412:T5)  [unwired: 9 in]
          n124 = call <vilib>:"WPI_MotorControlSetOutput.vi"("error in (no error)"=w411, "Output"=w415, "MotorControlDevRef"=w412) -> ()  [unwired: 6 in, 3 out]
          n125 = call <vilib>:"WPI_MotorControlSetOutput.vi"("error in (no error)"=w413, "Output"=w415, "MotorControlDevRef"=w414) -> ()  [unwired: 6 in, 3 out]
        }
        frame #1 {
          n126 = global write "MotorPositionGlobals.vi" "BallHolder"(FALSE ("BallHolder")) -> ()
        }
        frame #2 {
          n127 = Wait (ms)(milliseconds to wait=u32 700) -> ()  [unwired: 1 out]
        }
        frame #3 {
          n128 = call-poly <vilib>:"WPI_SolenoidSet.vi"("Value"=WPI_SolenoidValue."On", "SolenoidDevRef"=w425) -> ()  [unwired: 8 in, 2 out]
        }
        frame #4 {
          n129 = Wait (ms)(milliseconds to wait=u32 550) -> ()  [unwired: 1 out]
        }
        frame #5 {
          n130 = call-poly <vilib>:"WPI_SolenoidSet.vi"("Value"=WPI_SolenoidValue."Off", "SolenoidDevRef"=w429) -> ()  [unwired: 8 in, 2 out]
        }
        frame #6 {
          n131 = Wait (ms)(milliseconds to wait=u32 200) -> ()  [unwired: 1 out]
        }
        frame #7 {
        }
      }
      n132 = flat-sequence {
        tunnel: w396 -> [w403]
        tunnel: [w403] -> w394
        tunnel: [w405] -> w395
        tunnel: w394 -> [w405]
        tunnel: [w408] -> w393
        tunnel: w395 -> [w408]
        frame #0 {
          n133 = global write "MotorPositionGlobals.vi" "WinchSetpoint"(25.0 ("WinchPosition")) -> ()
        }
        frame #1 {
          n134 = call "WaitForWinchError.vi"("Timeout (ms)"=3000.0, "AllowedError"=40.0) -> ()  [unwired: 9 in, 1 out]
        }
        frame #2 {
          # "Fender Shot Default"
          n135 = global write "MotorPositionGlobals.vi" "TensionerSetpoint"(-90000.0 ("TensionerSetpoint")) -> ()
          n136 = global write "MotorPositionGlobals.vi" "WinchSetpoint"(4900.0 ("WinchPosition")) -> ()
        }
      }
    }
    frame "End" {
    }
  }
  "Terminate" <- w3
  n137 = feedback-in #1(w4) -> ()
